vi "Drive Axis Modifications.vi"(1 "Drive Info In":T1) -> (0 "Drive Info Out":T1)   [LabVIEW 2013]
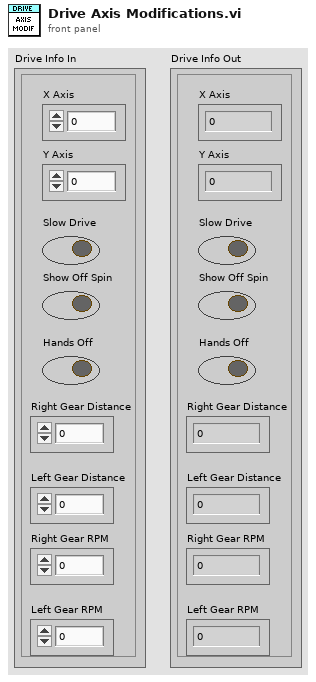
[diagram p1: front panel]
types:
  T1 = cluster{"X Axis":dbl, "Y Axis":dbl, "Slow Drive":bool, "Show Off Spin":bool, "Hands Off":bool, "Right Gear Distance":dbl, "Left Gear Distance ":dbl, "Right Gear RPM":dbl, "Left Gear RPM":dbl}
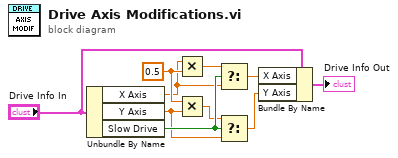
[diagram p0: block diagram]
diagram:
  w7 = 0.5 ("y")
  n1 = Unbundle By Name("Drive Info In") -> ("X Axis"=w2:dbl, "Y Axis"=w1:dbl, "Slow Drive"=w8:bool)
  n2 = Multiply(x=w2, y=w7) -> (x*y=w6:dbl)
  n3 = Multiply(x=w7, y=w1) -> (x*y=w3:dbl)
  n4 = Select(t=w6, s=w8, f=w2) -> (s? t:f=w5:dbl)
  n5 = Select(t=w3, s=w8, f=w1) -> (s? t:f=w4:dbl)
  n6 = Bundle By Name(cluster="Drive Info In", "X Axis"=w5, "Y Axis"=w4) -> (→"Drive Info Out":T1)
